vi "ABB Report Heat Run.vi"(10 "Report in":string, 11 "Heat run #":i32) -> (2 "Report out":string)   [LabVIEW 2017]
uses:
  ABB global.vi
panel:
  out "appended array":string[][](array[string])
  out "subarray":dbl[](array[numeric])
  out "Heat run":cluster{"Heat run results":dbl[], dbl[]}[](graph)
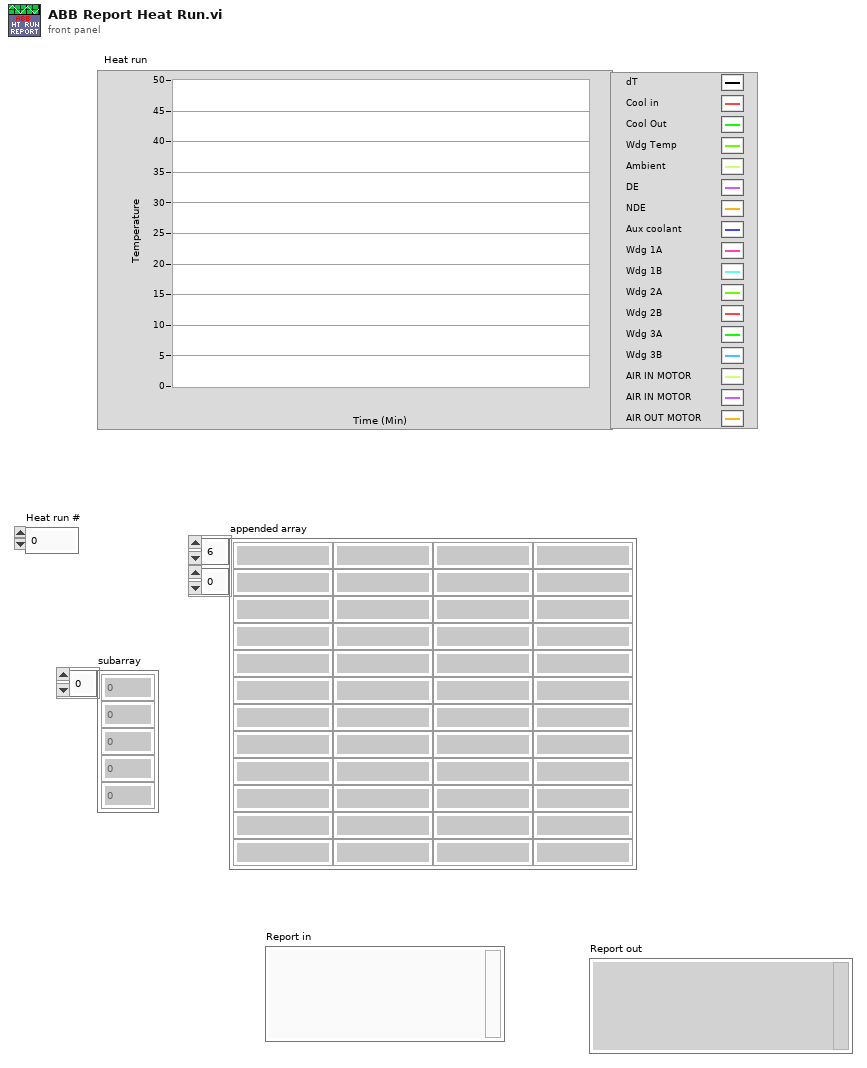
[diagram p1: front panel]
types:
  T1 = cluster{"temp. alloc":i32[], "category":i32[], "Category names":string[], "Category none names":string[]}
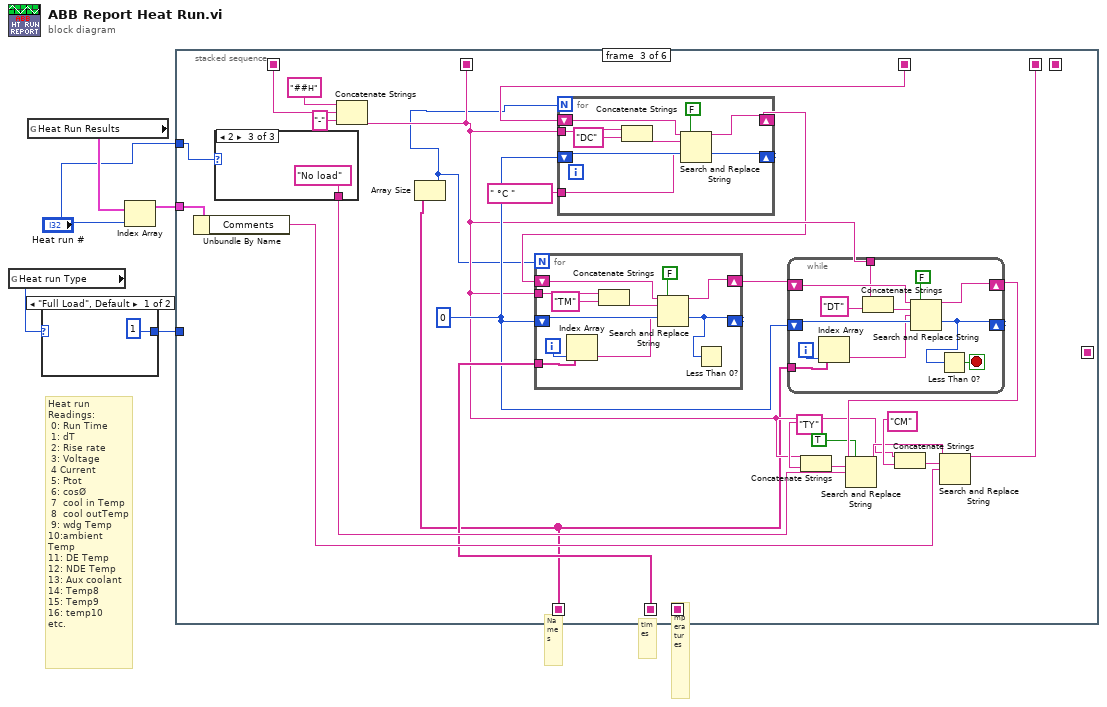
[diagram p0: block diagram]
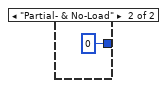
[diagram p2: hidden frame]
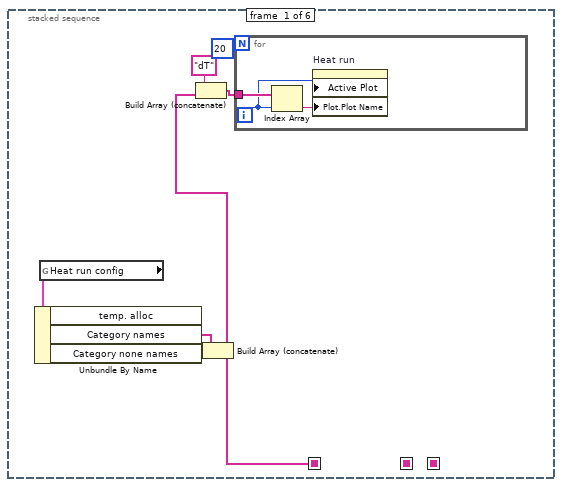
[diagram p3: hidden frame]
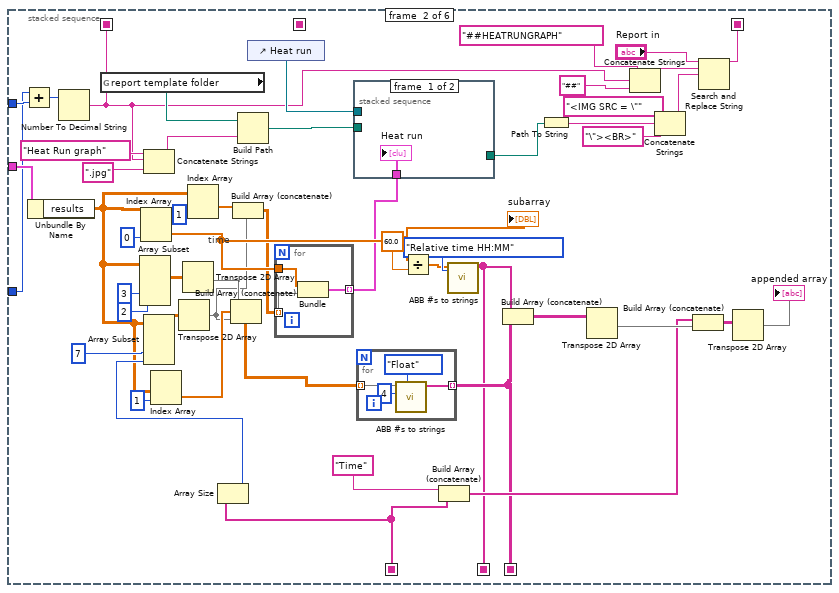
[diagram p4: hidden frame]
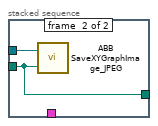
[diagram p5: hidden frame]
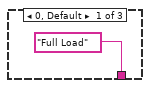
[diagram p6: hidden frame]
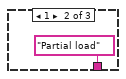
[diagram p7: hidden frame]
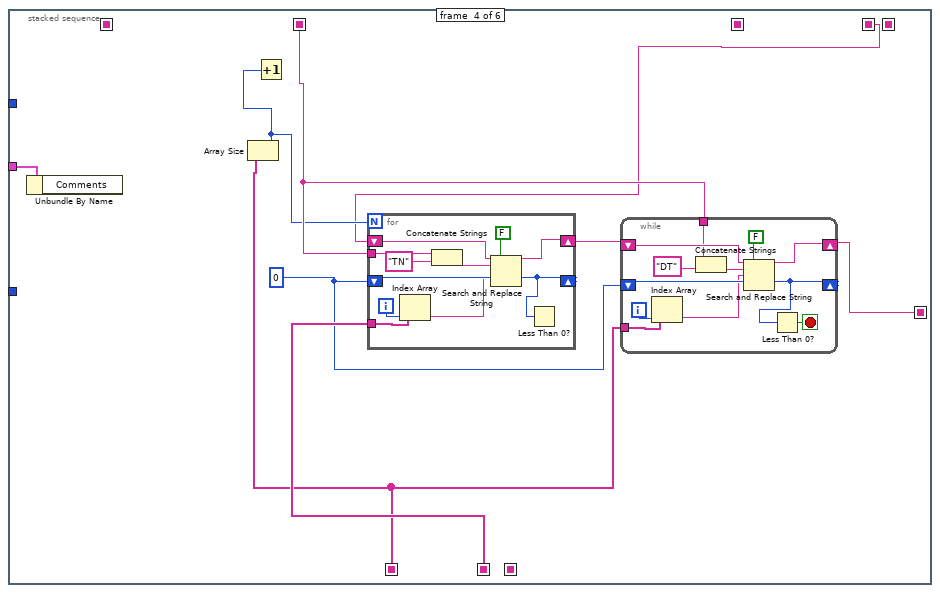
[diagram p8: hidden frame]
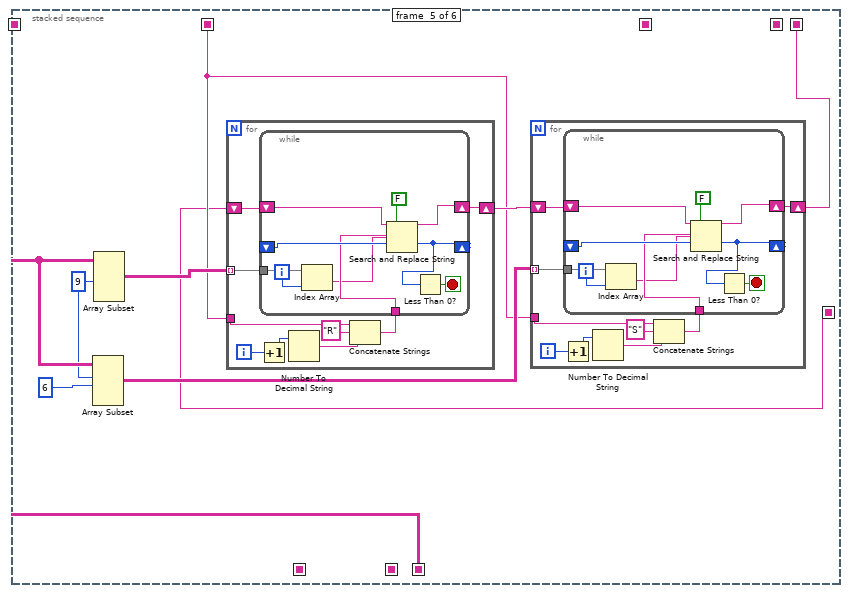
[diagram p9: hidden frame]
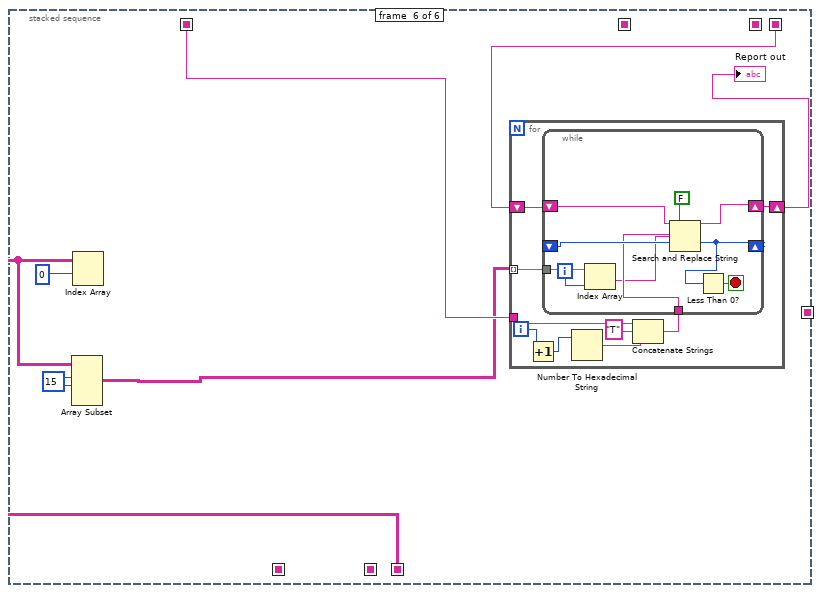
[diagram p10: hidden frame]
diagram:
  # "Heat run Readings:\n 0: Run Time\n 1: dT\n 2: Rise rate\n 3: Voltage\n 4 Current\n 5: Ptot\n 6: cosØ\n 7  cool in Temp\n 8  cool outTemp\n 9: wdg Temp\n10:ambient Temp\n11: DE Temp\n12: NDE Temp\n13: Aux coolant\n14: Temp8\n15: Temp9\n16: temp10\netc."
  # "Names"
  # "Temperatures"
  # "times"
  n1 = global read "ABB global.vi" "Heat run Type"() -> (w2:enum16{"Full Load", "Partial- & No-Load"})
  n2 = global read "ABB global.vi" "Heat Run Results"() -> (w4:cluster{"results":dbl[][], "Comments":string}[])
  n3 = case shown="\"Full Load\", Default" w2 {
    tunnel: [1 0] -> w1
    frame "Full Load", Default {
    }
    frame "Partial- & No-Load" {
    }
  }
  n4 = Index Array(array=w4, index="Heat run #") -> (element=w5:cluster{"results":dbl[][], "Comments":string})
  n5 = stacked-sequence {
    seq-local: [_ w60 _ _ _ _] -> [_ _ w83 _ _ _]
    seq-local: [_ w54 _ _ _ _] -> [_ _ _ _ w176 w223]
    seq-local: [w8 _ _ _ _ _] -> [_ w31 w82 w142 _ _]
    seq-local: [_ w53 _ _ _ _] -> [_ _ w89 w145 _ _]
    seq-local: [_ w40 _ _ _ _] -> [_ _ w101 _ _ _]
    seq-local: [_ _ w88 _ _ _] -> [_ _ _ w138 _ _]
    seq-local: [_ _ w86 _ _ _] -> [_ _ _ w143 w173 w222]
    seq-local: [_ _ _ w139 _ _] -> [_ _ _ _ w172 _]
    seq-local: [_ _ _ _ w171 _] -> [_ _ _ _ _ w219]
    tunnel: w5 -> [_ w59 w99 w146 _ _]
    tunnel: "Heat run #" -> [_ w52 w92 _ _ _]
    tunnel: w1 -> [_ w38 _ _ _ _]
    frame #0 {
      n6 = global read "ABB global.vi" "Heat run config"() -> (w9:T1)
      n7 = Unbundle By Name(w9) -> ("Category names"=w11:string[], "Category none names"=w10:string[])  [unwired: 1 out]
      n8 = Build Array (concatenate)(w11, w10) -> (w8:string[])
      n9 = Build Array (concatenate)("dT", w8) -> (w13:string[])
      n10 = for {
        N: 20 -> [_]
        tunnel: w13 -> [w17]
        i -> [w16]
        n11 = Index Array(array=w17, index=w16) -> (element=w15:string)
        n12 = property on="Heat run" class="XYGraph (strict)"("Active Plot"=w16, "Plot.Plot Name"=w15) -> ()  [unwired: 2 in, 2 out]
      }
    }
    frame #1 {
      # "time"
      n13 = Add(x=w38, y=w52) -> (x+y=w51:i32)
      n14 = Unbundle By Name(w59) -> ("results"=w22:dbl[][])
      n15 = Number To Decimal String(number=w51) -> (decimal integer string=w40:string)  [unwired: 1 in]
      n16 = global read "ABB global.vi" "report template folder"() -> (w61:path)
      n17 = Array Subset(array=w22, index (col)=3 ("index"), length (col)=2 ("length")) -> (w27:dbl[][])  [unwired: 2 in]
      n18 = Index Array(array=w22, index (col)=0 ("disabled index (col)")) -> (element=w35:dbl[])  [unwired: 1 in]
      "subarray" <- w35
      n19 = Concatenate Strings("Heat Run graph" ("name or relative path"), w40, ".jpg" ("name or relative path")) -> (w46:string)
      n20 = Index Array(array=w22, index (col)=1 ("disabled index (col)")) -> (element=w24:dbl[])  [unwired: 1 in]
      n21 = Transpose 2D Array(2D array=w27) -> (transposed array=w26:dbl[][])
      n22 = Index Array(array=w22, index (col)=1 ("disabled index (col)")) -> (element=w20:dbl[])  [unwired: 1 in]
      n23 = Array Size(array=w31) -> (size(s)=w30:i32)
      n24 = Array Subset(array=w22, index (col)=7 ("index"), length (col)=w30) -> (w43:dbl[][])  [unwired: 2 in]
      n25 = Transpose 2D Array(2D array=w43) -> (transposed array=w19:dbl[][])
      n26 = Build Array (concatenate)(w26, w24, w19) -> (w23:dbl[][])
      n27 = Build Array (concatenate)(w20, w19) -> (w18:dbl[][])
      n28 = Build Path(base path=w61, name or relative path=w46) -> (appended path=w64:path)
      n29 = control-ref of="Heat run"() -> (w68:refnum<vi>)
      n30 = for {
        tunnel: w35 -> [w78]
        tunnel: w18 -> [w77] mode=indexing
        tunnel: [w76] -> w33 mode=indexing
        n31 = Bundle("results"=w78, w77) -> (w76:cluster{"results":dbl[], dbl[]})  [unwired: 1 in]
      }
      n32 = stacked-sequence {
        tunnel: w68 -> [_ w71]
        tunnel: w64 -> [_ w70]
        tunnel: w33 -> [w69 _]
        tunnel: [_ w70] -> w32
        frame #0 {
          "Heat run" <- w69
        }
        frame #1 {
          n33 = call "ABB SaveXYGraphImage_JPEG.vi"("Path"=w70, "COntrolReference"=w71) -> ()  [unwired: 2 in]
        }
      }
      n34 = for {
        tunnel: w23 -> [w75] mode=indexing
        tunnel: [w72] -> w54 mode=indexing
        n35 = call "ABB #s to strings.vi"("# type"=enum16{"Float", "Relative time HH:MM"}."Float", "Precision"=4, "Numbers in"=w75) -> ("Strings out"=w72:string[])  [unwired: 8 in]
      }
      n36 = Divide(x=w35, y=60.0 ("Numeric")) -> (x/y=w36:dbl[])
      n37 = Build Array (concatenate)("Time", w31) -> (w55:string[])
      n38 = call "ABB #s to strings.vi"("# type"=enum16{"Float", "Relative time HH:MM"}."Relative time HH:MM", "Numbers in"=w36) -> ("Strings out"=w53:string[])  [unwired: 9 in]
      n39 = Build Array (concatenate)(w53, w54) -> (w41:string[][])
      n40 = Path To String(path=w32) -> (string=w63:string)
      n41 = Transpose 2D Array(2D array=w41) -> (transposed array=w58:string[][])
      n42 = Concatenate Strings("##HEATRUNGRAPH", w40, "##") -> (w39:string)
      n43 = Concatenate Strings("<IMG SRC = \"", w63, "\"><BR>" ("string")) -> (w65:string)
      n44 = Build Array (concatenate)(w55, w58) -> (w57:string[][])
      n45 = Search and Replace String(input string="Report in", search string=w39, replace string=w65) -> (result string=w60:string)  [unwired: 5 in, 3 out]
      n46 = Transpose 2D Array(2D array=w57) -> (transposed array=→"appended array":string[][])
    }
    frame #2 {
      w87 = 0 ("offset past replacement")
      n47 = Unbundle By Name(w99) -> ("Comments"=w93:string)
      n48 = case shown="2" w92 {
        tunnel: ["Full Load" "Partial load" "No load"] -> w91
        frame 0, Default {
        }
        frame 1 {
        }
        frame 2 {
        }
      }
      n49 = Concatenate Strings("##H" ("search string"), w101, "-" ("string")) -> (w86:string)
      n50 = Array Size(array=w82) -> (size(s)=w79:i32)
      n51 = for {
        N: w79 -> [_]
        shift-right: [w121] -> w84
        shift-left: w83 -> [w122]
        shift-right: [w114] -> _
        shift-left: w87 -> [w120]
        tunnel: w86 -> [w118]
        tunnel: " °C " ("Unit") -> [w115]
        n52 = Concatenate Strings(w118, "DC" ("search string")) -> (w116:string)
        n53 = Search and Replace String(replace all?=FALSE ("replace all? (F)"), input string=w122, search string=w116, replace string=w115, offset=w120) -> (result string=w121:string, offset past replacement=w114:i32)  [unwired: 3 in, 2 out]
      }
      n54 = for {
        N: w79 -> [_]
        shift-right: [w112] -> w80
        shift-left: w84 -> [w113]
        tunnel: w89 -> [w108]
        shift-right: [w109] -> _
        shift-left: w87 -> [w111]
        tunnel: w86 -> [w106]
        i -> [w107]
        n55 = Index Array(array=w108, index=w107) -> (element=w103:string)
        n56 = Concatenate Strings(w106, "TM" ("search string")) -> (w104:string)
        n57 = Search and Replace String(replace all?=FALSE ("replace all? (F)"), input string=w113, search string=w104, replace string=w103, offset=w111) -> (result string=w112:string, offset past replacement=w109:i32)  [unwired: 3 in, 2 out]
        n58 = Less Than 0?(x=w109) -> ()  [unwired: 1 out]
      }
      n59 = while {
        shift-right: [w136] -> w90
        shift-left: w80 -> [w137]
        tunnel: w82 -> [w131]
        shift-right: [w132] -> _
        shift-left: w87 -> [w135]
        tunnel: w86 -> [w129]
        i -> [w130]
        stop <- w133 stop-if-true
        n60 = Index Array(array=w131, index=w130) -> (element=w126:string)
        n61 = Concatenate Strings(w129, "DT" ("search string")) -> (w127:string)
        n62 = Search and Replace String(replace all?=FALSE ("replace all? (F)"), input string=w137, search string=w127, replace string=w126, offset=w135) -> (result string=w136:string, offset past replacement=w132:i32)  [unwired: 3 in, 2 out]
        n63 = Less Than 0?(x=w132) -> (x < 0?=w133:bool)
      }
      n64 = Concatenate Strings(w86, "TY" ("search string")) -> (w98:string)
      n65 = Search and Replace String(replace all?=TRUE ("replace all? (F)"), input string=w90, search string=w98, replace string=w91) -> (result string=w94:string)  [unwired: 4 in, 3 out]
      n66 = Concatenate Strings(w86, "CM" ("search string")) -> (w95:string)
      n67 = Search and Replace String(input string=w94, search string=w95, replace string=w93) -> (result string=w88:string)  [unwired: 5 in, 3 out]
    }
    frame #3 {
      w144 = 0 ("offset past replacement")
      n68 = Unbundle By Name(w146) -> ()  [unwired: 1 out]
      n69 = Array Size(array=w142) -> (size(s)=w141:i32)
      n70 = Increment(x=w141) -> ()  [unwired: 1 out]
      n71 = for {
        N: w141 -> [_]
        shift-right: [w156] -> w140
        shift-left: w138 -> [w157]
        tunnel: w145 -> [w152]
        shift-right: [w153] -> _
        shift-left: w144 -> [w155]
        tunnel: w143 -> [w150]
        i -> [w151]
        n72 = Index Array(array=w152, index=w151) -> (element=w147:string)
        n73 = Concatenate Strings(w150, "TN" ("search string")) -> (w148:string)
        n74 = Search and Replace String(replace all?=FALSE ("replace all? (F)"), input string=w157, search string=w148, replace string=w147, offset=w155) -> (result string=w156:string, offset past replacement=w153:i32)  [unwired: 3 in, 2 out]
        n75 = Less Than 0?(x=w153) -> ()  [unwired: 1 out]
      }
      n76 = while {
        shift-right: [w168] -> w139
        shift-left: w140 -> [w169]
        tunnel: w142 -> [w163]
        shift-right: [w164] -> _
        shift-left: w144 -> [w167]
        tunnel: w143 -> [w161]
        i -> [w162]
        stop <- w165 stop-if-true
        n77 = Index Array(array=w163, index=w162) -> (element=w158:string)
        n78 = Concatenate Strings(w161, "DT" ("search string")) -> (w159:string)
        n79 = Search and Replace String(replace all?=FALSE ("replace all? (F)"), input string=w169, search string=w159, replace string=w158, offset=w167) -> (result string=w168:string, offset past replacement=w164:i32)  [unwired: 3 in, 2 out]
        n80 = Less Than 0?(x=w164) -> (x < 0?=w165:bool)
      }
    }
    frame #4 {
      w175 = 9 ("length")
      n81 = Array Subset(array=w176, index (row)=w175, length (row)=6 ("length")) -> (w174:string[][])  [unwired: 2 in]
      n82 = Array Subset(array=w176, length (row)=w175) -> (w177:string[][])  [unwired: 3 in]
      n83 = for {
        tunnel: w177 -> [w206] mode=indexing
        shift-right: [w204] -> w178
        shift-left: w172 -> [w205]
        tunnel: w173 -> [w199]
        i -> [w203]
        n84 = Increment(x=w203) -> (x+1=w202:i32)
        n85 = Number To Decimal String(number=w202) -> (decimal integer string=w200:string)  [unwired: 1 in]
        n86 = Concatenate Strings(w199, "R" ("search string"), w200) -> (w198:string)
        n87 = while {
          shift-right: [w215] -> w204
          shift-left: w205 -> [w216]
          shift-right: [w211] -> _
          shift-left: _ -> [w214]
          tunnel: w206 -> [w209]
          tunnel: w198 -> [w208]
          i -> [w210]
          stop <- w212 stop-if-true
          n88 = Index Array(array=w209, index=w210) -> (element=w207:string)
          n89 = Search and Replace String(replace all?=FALSE ("replace all? (F)"), input string=w216, search string=w208, replace string=w207, offset=w214) -> (result string=w215:string, offset past replacement=w211:i32)  [unwired: 3 in, 2 out]
          n90 = Less Than 0?(x=w211) -> (x < 0?=w212:bool)
        }
      }
      n91 = for {
        tunnel: w174 -> [w187] mode=indexing
        shift-right: [w185] -> w171
        shift-left: w178 -> [w186]
        tunnel: w173 -> [w180]
        i -> [w184]
        n92 = Increment(x=w184) -> (x+1=w183:i32)
        n93 = Number To Decimal String(number=w183) -> (decimal integer string=w181:string)  [unwired: 1 in]
        n94 = Concatenate Strings(w180, "S" ("search string"), w181) -> (w179:string)
        n95 = while {
          shift-right: [w196] -> w185
          shift-left: w186 -> [w197]
          shift-right: [w192] -> _
          shift-left: _ -> [w195]
          tunnel: w187 -> [w190]
          tunnel: w179 -> [w189]
          i -> [w191]
          stop <- w193 stop-if-true
          n96 = Index Array(array=w190, index=w191) -> (element=w188:string)
          n97 = Search and Replace String(replace all?=FALSE ("replace all? (F)"), input string=w197, search string=w189, replace string=w188, offset=w195) -> (result string=w196:string, offset past replacement=w192:i32)  [unwired: 3 in, 2 out]
          n98 = Less Than 0?(x=w192) -> (x < 0?=w193:bool)
        }
      }
    }
    frame #5 {
      w220 = 15 ("index")
      n99 = Array Subset(array=w223, index (row)=w220, length (row)=w220) -> (w217:string[][])  [unwired: 2 in]
      n100 = Index Array(array=w223, index (row)=0 ("length")) -> ()  [unwired: 1 in, 1 out]
      n101 = for {
        tunnel: w217 -> [w232] mode=indexing
        shift-right: [w230] -> w221
        shift-left: w219 -> [w231]
        tunnel: w222 -> [w225]
        i -> [w229]
        n102 = Increment(x=w229) -> (x+1=w228:i32)
        n103 = Number To Hexadecimal String(2:w228) -> (0:w226:string)  [unwired: 1 in]
        n104 = Concatenate Strings(w225, "T" ("search string"), w226) -> (w224:string)
        n105 = while {
          shift-right: [w241] -> w230
          shift-left: w231 -> [w242]
          shift-right: [w237] -> _
          shift-left: _ -> [w240]
          tunnel: w232 -> [w235]
          tunnel: w224 -> [w234]
          i -> [w236]
          stop <- w238 stop-if-true
          n106 = Index Array(array=w235, index=w236) -> (element=w233:string)
          n107 = Search and Replace String(replace all?=FALSE ("replace all? (F)"), input string=w242, search string=w234, replace string=w233, offset=w240) -> (result string=w241:string, offset past replacement=w237:i32)  [unwired: 3 in, 2 out]
          n108 = Less Than 0?(x=w237) -> (x < 0?=w238:bool)
        }
      }
      "Report out" <- w221
    }
  }
